vi "Read Update Events.vi"(8 "error in (no error)":errorcluster, 11 "CS++SimMotor in":refnum<class "CS++SimMotor.lvclass">) -> (0 "error out":errorcluster, 2 "Update Events":T1, 3 "CS++SimMotor out":refnum<class "CS++SimMotor.lvclass">)   [LabVIEW 2015, in "CS++SimMotor.lvlib" / "CS++SimMotor.lvclass"]
uses:
  CS++SimMotor.lvclass
  CS++SimMotor.lvclass/CS++SimMotor.ctl
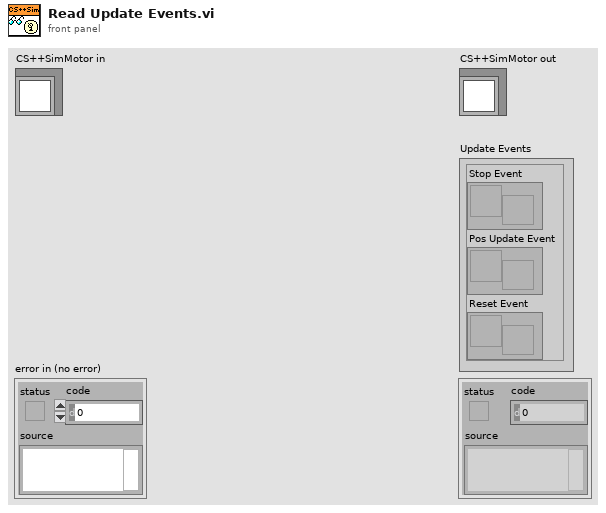
[diagram p1: front panel]
types:
  T1 = cluster{"Stop Event":refnum<user-event>, "Pos Update Event":refnum<user-event>, "Reset Event":refnum<user-event>}
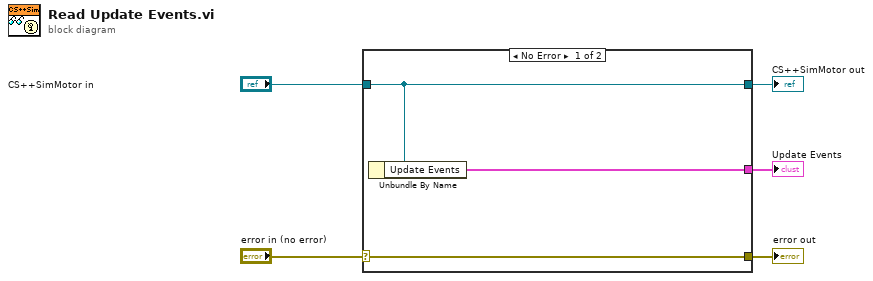
[diagram p0: block diagram]
diagram:
  n1 = case shown="No Error" "error in (no error)" {
    selector: "error in (no error)" -> [w8 w9]
    tunnel: [w8 w9] -> w4
    tunnel: [w7 w10] -> w2
    tunnel: "CS++SimMotor in" -> [w7 w10]
    tunnel: [w6 _] -> w1
    frame No Error {
      n2 = Unbundle By Name(w7) -> ("Update Events"=w6:T1)
    }
    frame Error {
    }
  }
  "error out" <- w4
  "CS++SimMotor out" <- w2
  "Update Events" <- w1
